vi "Getpinstatusresponse.vi"(8 "error in (no error)":errorcluster, 11 "NXP in":refnum<class "NXP.lvclass">) -> (0 "error out":errorcluster, 2 "Value":string, 3 "NXP out":refnum<class "NXP.lvclass">)   [LabVIEW 2019, in "NXP.lvclass"]
uses:
  NXP.lvclass
  NXP.lvclass/NXP.ctl
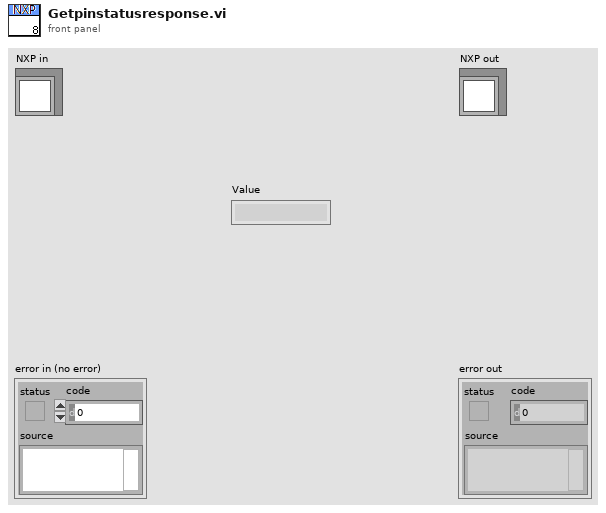
[diagram p1: front panel]
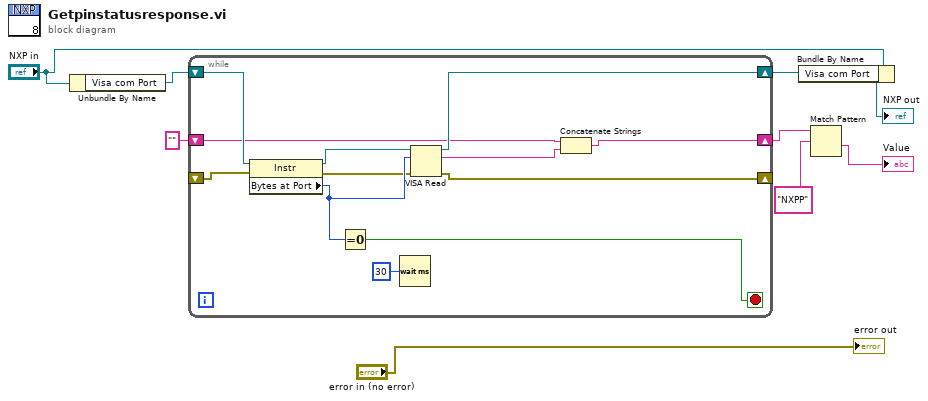
[diagram p0: block diagram]
diagram:
  n1 = Unbundle By Name("NXP in") -> ("Visa com Port"=w7:refnum<visa-resource-name>)
  n2 = while {
    shift-right: [w16] -> _
    shift-left: _ -> [w15]
    shift-right: [w14] -> w6
    shift-left: w7 -> [w21]
    shift-right: [w12] -> w4
    shift-left: "" -> [w13]
    stop <- w19 stop-if-true
    n3 = property class="Instr"(reference=w21, error in=w15) -> (reference out=w20:refnum<visa-resource-name>, error out=w17:errorcluster, "Bytes at Port"=w18:u32)
    n4 = Equal To 0?(x=w18) -> (x = 0?=w19:bool)
    n5 = Wait (ms)(milliseconds to wait=u32 30) -> ()  [unwired: 1 out]
    n6 = VISA Read(VISA resource name=w20, byte count=w18, error in (no error)=w17) -> (VISA resource name out=w14:refnum<visa-resource-name>, read buffer=w11:string, error out=w16:errorcluster)  [unwired: 1 out]
    n7 = Concatenate Strings(w13, w11) -> (w12:string)
  }
  n8 = Bundle By Name(cluster="NXP in", "Visa com Port"=w6) -> (→"NXP out":refnum<class "NXP.lvclass">)
  n9 = Match Pattern(string=w4, regular expression="NXPP") -> (after substring=→"Value":string)  [unwired: 1 in, 3 out]
  "error out" <- "error in (no error)"
